vi "sub_Exit.vi"(8 "error in":errorcluster caption="에러 입력", 11 "Wash Options":refnum<vi>) -> (0 "error out":errorcluster caption="에러 출력")   [LabVIEW 2018]
uses:
  Control/Wash Options.ctl
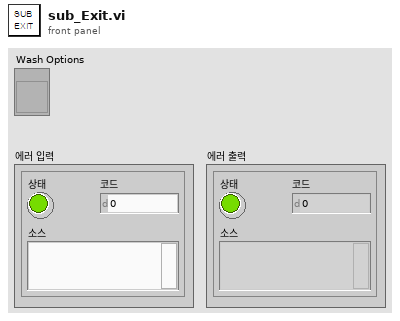
[diagram p1: front panel]
types:
  T1 = typedef "Wash Options.ctl" = cluster{"Under Body Wash":bool, "Bug Remover":bool, "Pre-Soak":bool, "High Pressure Wash":bool, "Low Pressure Wax":bool, "Spot Free Rinse":bool, "Tire Shine Foam":bool, "Air Dry":bool}
  T2 = enum8{"Enabled", "Disabled", "Disabled and Grayed Out"}
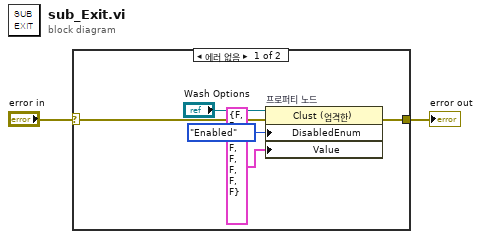
[diagram p0: block diagram]
diagram:
  n1 = case shown="에러 없음" "error in" {
    selector: "error in" -> [w6 w8]
    tunnel: [w7 w8] -> w1
    frame No Error {
      n2 = property on="프로퍼티 노드" class="Clust (엄격한)"(reference="Wash Options", error in=w6, "DisabledEnum"=T2."Enabled" ("비활성화"), "Value"=T1 {"Under Body Wash"=FALSE, "Bug Remover"=FALSE, "Pre-Soak"=FALSE, "High Pressure Wash"=FALSE, "Low Pressure Wax"=FALSE, "Spot Free Rinse"=FALSE, "Tire Shine Foam"=FALSE, "Air Dry"=FALSE} ("값")) -> (error out=w7:errorcluster)  [unwired: 1 out]
    }
    frame Error {
    }
  }
  "error out" <- w1
